vi "PID Calculate PID.vi"(0 "Error":dbl, 5 "Last Error":dbl, 7 "From Shift Register":dbl, 9 "Gains":cluster{"P":dbl, "I":dbl, "D":dbl}, 11 "Change in Time":u32) -> (4 "Output":dbl, 8 "To Shift Register":dbl)   [LabVIEW 2014]
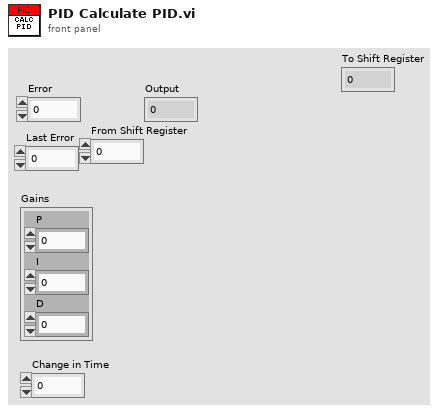
[diagram p1: front panel]
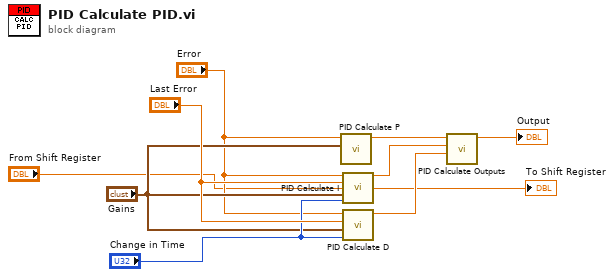
[diagram p0: block diagram]
diagram:
  n1 = call "PID Calculate P.vi"("Gains"="Gains", "Error"="Error") -> ("Output"=w3:dbl)  [unwired: 9 in]
  n2 = call "PID Calculate I.vi"("Error"="Error", "Last Error"="Last Error", "From Shift Register"="From Shift Register", "Gains"="Gains", "Change in Time"="Change in Time") -> ("Output"=w4:dbl, "To Shift Register"=→"To Shift Register":dbl)  [unwired: 9 in]
  n3 = call "PID Calculate D.vi"("Change in Time"="Change in Time", "Gains"="Gains", "Last Error"="Last Error", "Error"="Error") -> ("Output"=w6:dbl)  [unwired: 7 in]
  n4 = call "PID Calculate Outputs.vi"("D Output"=w6, "I Output"=w4, "P Output"=w3) -> ("Output"=→"Output":dbl)  [unwired: 8 in]
